vi "test - Remove Filter - 2.vi"(8 "error in (no error)":errorcluster, 11 "TestCase in":refnum<class "Remove Filter Unit Test.lvclass">) -> (0 "error out":errorcluster, 3 "TestCase out":refnum<class "Remove Filter Unit Test.lvclass">)   [LabVIEW 2016, in "Assert API Components.lvlib" / "Assert Display.lvlib" / "Main Display.lvlib" / "Remove Filter Unit Test.lvclass"]
uses:
  Remove Filter Unit Test.lvclass
  Remove Filter Unit Test.lvclass/Remove Filter Unit Test.ctl
  <vilib>/addons/_JKI Toolkits/VI Tester/TestCase.llb/TestCase.lvclass
  Core/Main Display/Main Display/Main Display.lvclass
  Core/Main Display/Main Display.lvlib
  C:/Program Files (x86)/National Instruments/LabVIEW 2016/vi.lib/addons/_JKI Toolkits/VI Tester/TestCase.llb/TestCase.lvclass
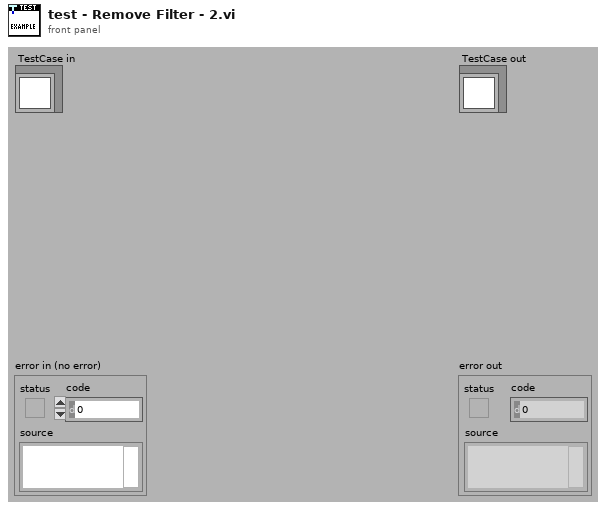
[diagram p1: front panel]
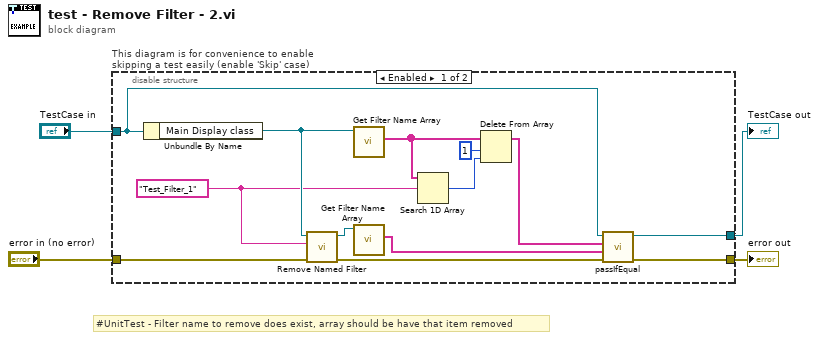
[diagram p0: block diagram]
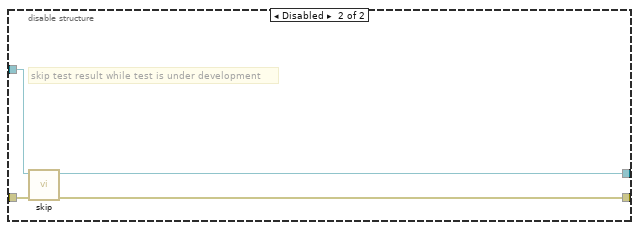
[diagram p2: hidden frame]
diagram:
  # "#UnitTest - Filter name to remove does exist, array should be have that item removed"
  n1 = disable-structure "This diagram is for convenience to enable skipping a test easily (enable 'Skip' case)" shown="Enabled" {
    disable-tunnel: "TestCase in" -> [w15 w21]
    disable-tunnel: [w17 w19] -> w1
    disable-tunnel: [w16 w20] -> w3
    disable-tunnel: "error in (no error)" -> [w13 w18]
    frame Enabled {
      w9 = "Test_Filter_1" ("Filter Name")
      n2 = Unbundle By Name(w15) -> ("Main Display class"=w10:refnum<class "Main Display.lvclass">)
      n3 = call "Remove Named Filter.vi"("error in (no error)"=w13, "Filter Name"=w9, "Main Display in"=w10) -> ("error out"=w12:errorcluster, "Main Display out"=w14:refnum<class "Main Display.lvclass">)  [unwired: 7 in]
      n4 = call "Get Filter Name Array.vi"("Main Display in"=w10) -> ("Filter Name Array"=w8:string[])  [unwired: 10 in]
      n5 = call "Get Filter Name Array.vi"("Main Display in"=w14) -> ("Filter Name Array"=w11:string[])  [unwired: 10 in]
      n6 = Search 1D Array(1D array=w8, element=w9) -> (index of element=w6:i32)  [unwired: 1 in]
      n7 = Delete From Array(array=w8, length=1, index=w6) -> (array with subset deleted=w5:string[])  [unwired: 1 out]
      n8 = call-dynamic "passIfEqual.vi"("error in (no error)"=w12, "y"=w11, "x"=w5, "TestCase in"=w15) -> ("error out"=w16:errorcluster, "TestCase out"=w17:refnum<class "Remove Filter Unit Test.lvclass">)  [unwired: 6 in]
    }
    frame Disabled {
      # "skip test result while test is under development"
      n9 = call <vilib>:"skip.vi"("error in (no error)"=w18, "TestCase in"=w21) -> ("error out"=w20:errorcluster, "TestCase out"=w19:refnum<class "Remove Filter Unit Test.lvclass">)  [unwired: 8 in]
    }
  }
  "error out" <- w3
  "TestCase out" <- w1
